vi "Polar Plot - Scale label.vi"(9 "grid measurements":T1, 10 "scale specs":cluster{"coordinate":i16, "label":string}[](array[cluster]), 11 "picture":picture) -> (3 "new picture":picture)   [LabVIEW 2020]
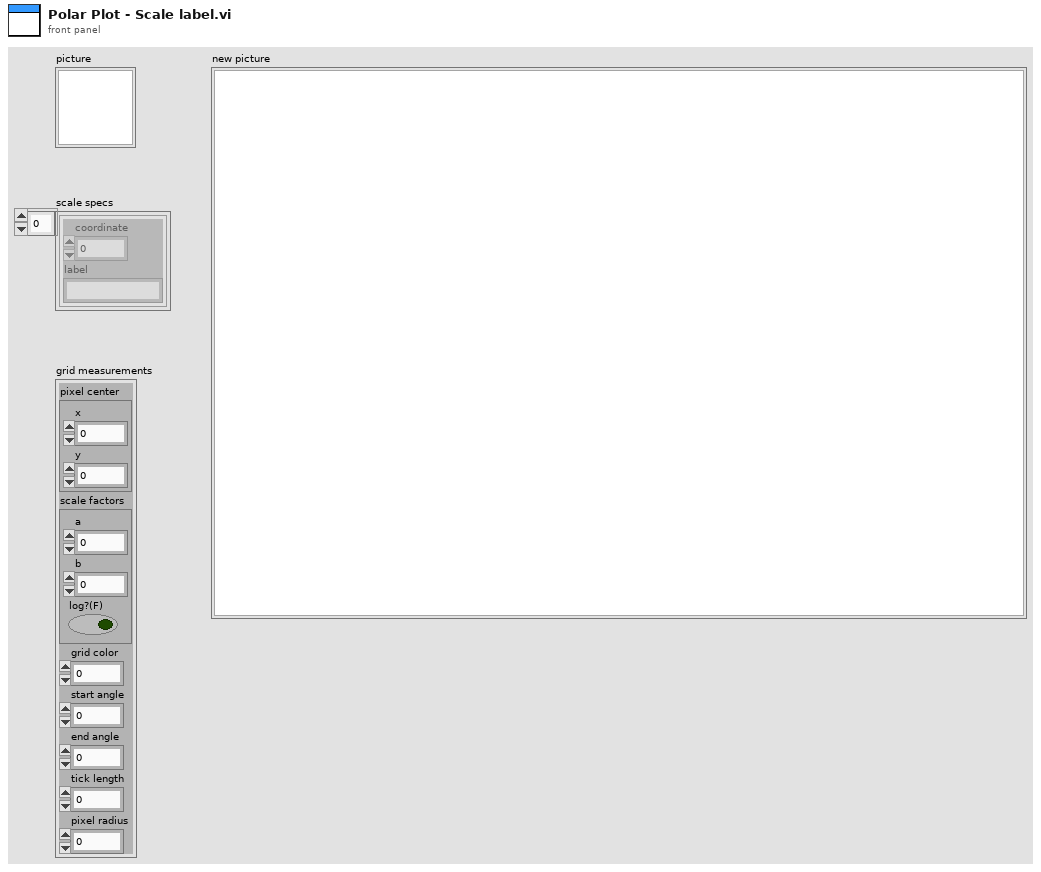
[diagram p1: front panel]
types:
  T1 = cluster{"pixel center":cluster{"x":i16, "y":i16}, "scale factors":cluster{"a":dbl, "b":dbl, "log?(F)":bool}, "grid color":u32, "start angle":dbl, "end angle":dbl, "tick length":i16, "pixel radius":i32}
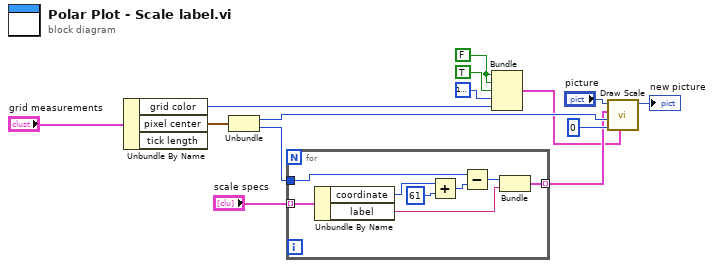
[diagram p0: block diagram]
diagram:
  w9 = FALSE
  n1 = Unbundle By Name("grid measurements") -> ("grid color"=w6:u32, "pixel center"=w4:cluster{"x":i16, "y":i16})  [unwired: 1 out]
  n2 = Unbundle(w4) -> ("x"=w11:i16, "y"=w5:i16)
  n3 = for {
    tunnel: "scale specs" -> [w22] mode=indexing
    tunnel: w5 -> [w20]
    tunnel: [w19] -> w2 mode=indexing
    n4 = Unbundle By Name(w22) -> ("coordinate"=w16:i16, "label"=w21:string)
    n5 = Add(x=w16, y=i16 61) -> (x+y=w17:i16)
    n6 = Subtract(x=w20, y=w17) -> (x-y=w18:i16)
    n7 = Bundle(w18, "label"=w21) -> (w19:cluster{i16, "label":string})  [unwired: 1 in]
  }
  n8 = Bundle(w9, w9, TRUE, u32 16777216, "grid color"=w6) -> (w1:cluster{bool, bool, bool, u32, "grid color":u32})  [unwired: 1 in]
  n9 = call <vilib>:"Draw Scale.vi"("scale attributes"=w1, "tick length(3)"=i16 0, "constant coordinate"=w11, "scale specs"=w2, "picture"="picture") -> ("new picture"=→"new picture":picture)  [unwired: 6 in]
